vi "GFITS_ImCreate.vi"(0 "logfile":path, 1 "hdrfile":path, 2 "amplifiers":u64, 3 "imageStruct":T1={"name"="/home/bonati/images/mono022", "Path"=path "", "bitpix"=16, "naxis"=2, "naxes"=[2224, 2048], "datatype"=0, "multiple extensions"=FALSE, "hdutype"=0, "writeToDisk"=TRUE, "num_of_ext"=0, "file ref"=0, "createnewimage"=TRUE}, 4 "error in (no error)":errorcluster, 7 "readmode":string, 8 "headers":bool=TRUE, 9 "imagesize(bytes)":i32, 10 "Database RefNum in":T2, 11 "def_head_tim":string="after", 12 "imretries":i32=20, 13 "m impath in":string) -> (5 "number of keywords":i32[](array[numeric]), 14 "file reference":u64, 15 "image name out":string, 16 "expID":string, 19 "error out":errorcluster)   [LabVIEW 2016]
uses:
  DBSHAND/private/vis/DatabaseHand_RefNum.ctl
  Common/public/vis/CMN_FVAR_action.ctl
  DBSHAND/private/vis/DatabaseHand_Element_Set(bool).vi
  DBSHAND/private/vis/DatabaseHand_Element_Get(bool).vi
  DBSHAND/private/vis/DatabaseHand_Element_Get(string).vi
  GFITS_Gbls.vi
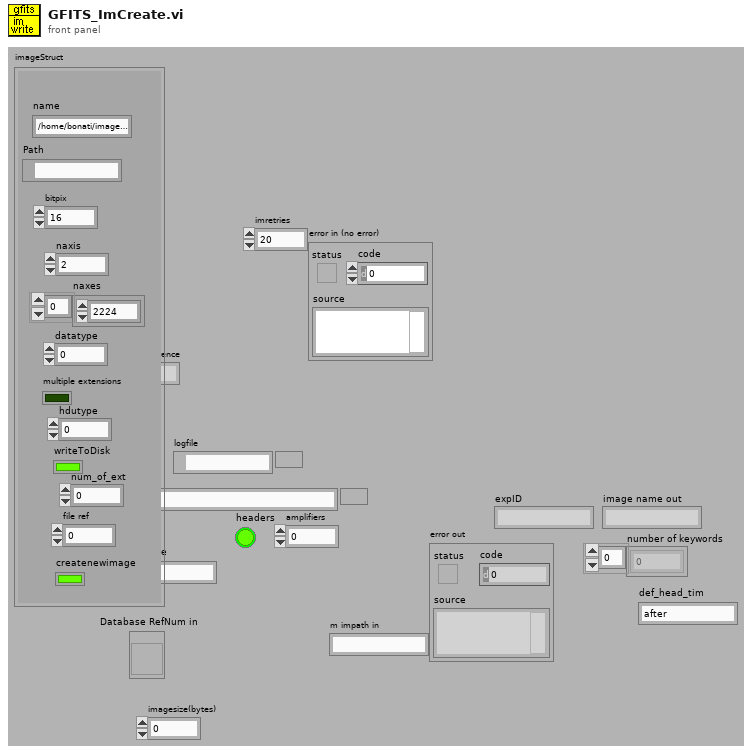
[diagram p1: front panel]
types:
  T1 = cluster{"name":string, "Path":path, "bitpix":i8, "naxis":u8, "naxes":u32[], "datatype":u16, "multiple extensions":bool, "hdutype":u16, "writeToDisk":bool, "num_of_ext":u8, "file ref":i32, "createnewimage":bool}
  T2 = typedef "DatabaseHand_RefNum.ctl" = refnum<vi>
  T3 = typedef "CMN_FVAR_action.ctl" = enum16{"read", "write"}
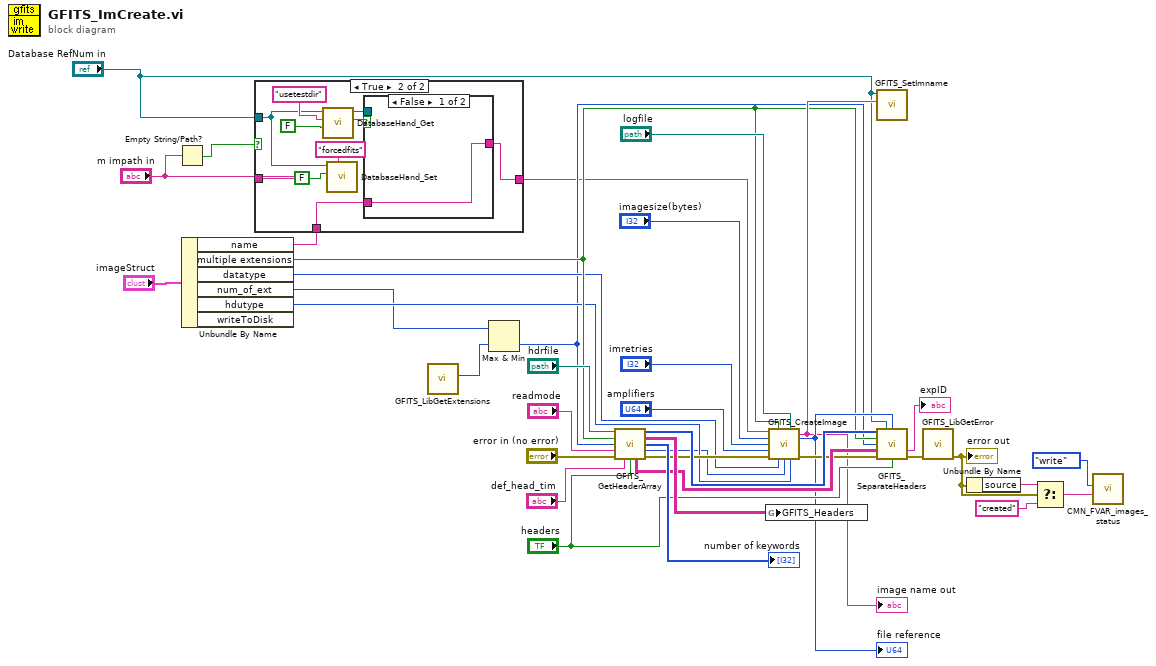
[diagram p0: block diagram]
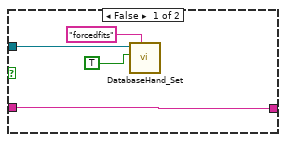
[diagram p2: hidden frame]
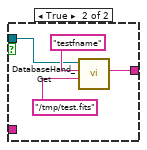
[diagram p3: hidden frame]
diagram:
  n1 = Empty String/Path?(string/path="m impath in") -> (empty?=w4:bool)
  n2 = Unbundle By Name("imageStruct") -> ("name"=w1:string, "multiple extensions"=w12:bool, "datatype"=w11:u16, "num_of_ext"=w8:u8, "hdutype"=w10:u16)  [unwired: 1 out]
  n3 = case shown="True" w4 {
    tunnel: "m impath in" -> [w39 _]
    tunnel: [w39 w50] -> w5
    tunnel: "Database RefNum in" -> [w41 w44]
    tunnel: w1 -> [_ w45]
    frame False {
      n4 = call-poly "DatabaseHand_Set.vi"("name"="forcedfits", "value"=TRUE, "Database RefNum in"=w41) -> ()  [unwired: 5 in, 4 out]
    }
    frame True {
      n5 = call-poly "DatabaseHand_Get.vi"("default value"=FALSE, "name"="usetestdir", "Database RefNum in"=w44) -> ("value"=w48:bool, "Database RefNum out"=w46:T2)  [unwired: 2 in, 5 out]
      n6 = call-poly "DatabaseHand_Set.vi"("name"="forcedfits", "value"=FALSE, "Database RefNum in"=w44) -> ()  [unwired: 5 in, 4 out]
      n7 = case shown="False" w48 {
        tunnel: [w51 w54] -> w50
        tunnel: w45 -> [w51 _]
        tunnel: w46 -> [_ w52]
        frame False {
        }
        frame True {
          n8 = call-poly "DatabaseHand_Get.vi"("default value"="/tmp/test.fits", "name"="testfname", "Database RefNum in"=w52) -> ("value"=w54:string)  [unwired: 2 in, 6 out]
        }
      }
    }
  }
  n9 = call "GFITS_LibGetExtensions.vi"() -> ("num extensions"=w7:i32)  [unwired: 2 in, 9 out]
  n10 = Max & Min(x=w8, y=w7) -> (min(x,y)=w6:i32)  [unwired: 1 out]
  n11 = call "GFITS_GetHeaderArray.vi"("file"="hdrfile", "mext"=w12, "number of Extensions"=w6, "readmode"="readmode", "error in (no error)"="error in (no error)", "def_timing"="def_head_tim", "headers"="headers") -> ("number of before"=w27:i32[], "After keys"=w29:string[][][], "number of after keywords"=→"number of keywords":i32[], "totkeys"=w9:i32, "before Keywords"=w26:string[][][], "error out"=w24:errorcluster)  [unwired: 3 out]
  n12 = global write "GFITS_Gbls.vi" "GFITS_Headers"(w29) -> ()
  n13 = call "GFITS_CreateImage.vi"("image name"=w5, "multiple extensions"=w12, "logfile"="logfile", "imagesize(bytes)"="imagesize(bytes)", "retries on error"="imretries", "amplifiers"="amplifiers", "error in (no error)"=w24, "datatype"=w11, "totkeys"=w9, "hdutype"=w10) -> ("image name out"=w17:string, "return value"=w22:u64, "error out"=w23:errorcluster)  [unwired: 3 out]
  "file reference" <- w22
  "image name out" <- w17
  n14 = call "GFITS_SetImname.vi"("name"=w17, "Database RefNum"="Database RefNum in") -> ()  [unwired: 1 in, 9 out]
  n15 = call "GFITS_SeparateHeaders.vi"("number of before keys"=w27, "Database RefNum in"="Database RefNum in", "ref"=w22, "mext"=w12, "number of Extensions"=w6, "Keywords"=w26, "error in (no error)"=w23, "headers"="headers") -> ("expID"=→"expID":string, "error out"=w16:errorcluster)  [unwired: 6 out]
  n16 = call "GFITS_LibGetError.vi"("error in (no error)"=w16) -> ("error out"=w15:errorcluster)  [unwired: 10 out]
  "error out" <- w15
  n17 = Unbundle By Name(w15) -> ("source"=w34:string)
  n18 = Select(t=w34, s=w15, f="created" ("value in")) -> (s? t:f=w33:string)
  n19 = call "CMN_FVAR_images_status.vi"("value in"=w33, "action"=CMN_FVAR_action."write") -> ()  [unwired: 9 out]
